vi "Calibration_Estimate X and Y Zoom voltages.vi"(11 "System Type":string="x.voltage") -> (2 "Y.ZOOM_estimated":dbl, 3 "X.ZOOM_estimated":dbl)   [LabVIEW 2012]
uses:
  Custom Controls and Typedefs/FGV_CalibrationKeyParams_Actions.ctl
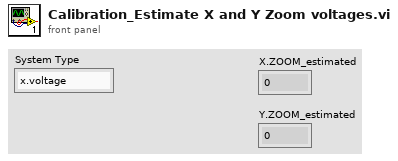
[diagram p1: front panel]
types:
  T1 = typedef "FGV_CalibrationKeyParams_Actions.ctl" = enum16{"Initialize", "Grab From SciScan and Store", "Read Parameters", "ReadGFGValue"}
  T2 = typedef "Calibration Key Param structure.ctl" = cluster{"GFG Variable Name":string, "Data Type":T3, "Value":variant}
  T3 = typedef "VariantType.lvlib/Type.ctl" = enum8{"Invalid Type", "Void", "I8", "I16", "I32", "I64", "U8", "U16", "U32", "U64", "Single Float", "Double Float", "Extended Float", "Single Complex", "Double Complex", "Extended Complex", "Enum U8", "Enum U16", "Enum U32", "Enum U64", "Single Float With Unit", "Double Float With Unit", "Extended Float With Unit", "Single Complex with Unit", "Double Complex with Unit", "Extended Complex with Unit", "Boolean", "String", "Path", "Picture", "Tag", "Array", "Cluster", "Variant", "LV Variant", "Waveform", "Timestamp", "Digital Waveform", "Digital Data", "ExpressData", "Refnum", "External Data", "VI", "Poly VI", "LabVIEW Class Instance", "Fixed Point"}
  T4 = cluster{"Key Parameters Array":T2[], "Key String":string}
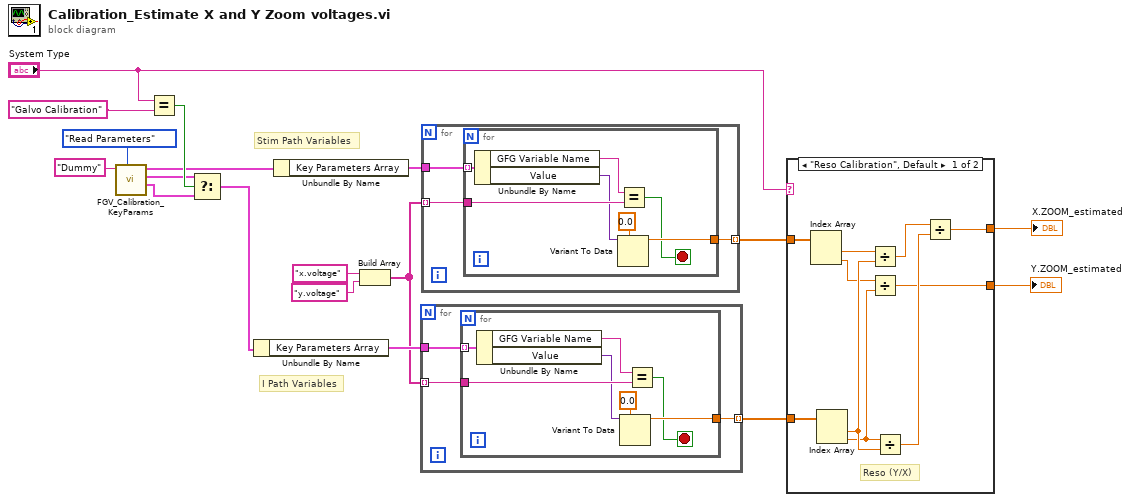
[diagram p0: block diagram]
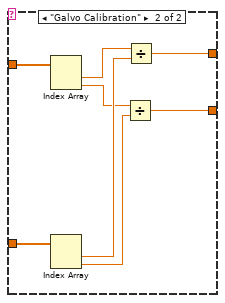
[diagram p2: hidden frame]
diagram:
  # "I Path Variables"
  # "Stim Path Variables"
  n1 = call "FGV_Calibration_KeyParams.vi"("Action"=FGV_CalibrationKeyParams_Actions."Read Parameters", "System Type"="Dummy") -> ("Imaging Reso Key Parameters"=w12:T4, "Imaging Galvo Key Parameters"=w13:T4, "Stimulating Galvo Key Parameters"=w5:T4)  [unwired: 4 in, 3 out]
  n2 = Equal?(x="System Type", y="Galvo Calibration" ("System Type")) -> (x = y?=w16:bool)
  n3 = Select(t=w13, s=w16, f=w12) -> (s? t:f=w6:T4)
  n4 = Unbundle By Name(w6) -> ("Key Parameters Array"=w8:T2[])
  n5 = Unbundle By Name(w5) -> ("Key Parameters Array"=w9:T2[])
  n6 = Build Array("x.voltage" ("System Type"), "y.voltage" ("System Type")) -> (w7:string[])
  n7 = for {
    tunnel: w7 -> [w20] mode=indexing
    tunnel: w8 -> [w21]
    tunnel: [w19] -> w3 mode=indexing
    n8 = for {
      tunnel: w21 -> [w28] mode=indexing
      tunnel: w20 -> [w27]
      tunnel: [w23] -> w19
      stop <- w22 stop-if-true
      n9 = Unbundle By Name(w28) -> ("GFG Variable Name"=w24:string, "Value"=w26:variant)
      n10 = Variant To Data(type=0.0, Variant=w26) -> (data=w23:dbl)  [unwired: 1 in, 1 out]
      n11 = Equal?(x=w24, y=w27) -> (x = y?=w22:bool)
    }
  }
  n12 = for {
    tunnel: w7 -> [w30] mode=indexing
    tunnel: w9 -> [w31]
    tunnel: [w29] -> w4 mode=indexing
    n13 = for {
      tunnel: w31 -> [w38] mode=indexing
      tunnel: w30 -> [w37]
      tunnel: [w33] -> w29
      stop <- w32 stop-if-true
      n14 = Unbundle By Name(w38) -> ("GFG Variable Name"=w34:string, "Value"=w36:variant)
      n15 = Variant To Data(type=0.0, Variant=w36) -> (data=w33:dbl)  [unwired: 1 in, 1 out]
      n16 = Equal?(x=w34, y=w37) -> (x = y?=w32:bool)
    }
  }
  n17 = case shown="\"Reso Calibration\", Default" "System Type" {
    tunnel: [w42 w52] -> w18
    tunnel: [w41 w51] -> w17
    tunnel: w4 -> [w40 w50]
    tunnel: w3 -> [w39 w49]
    frame "Reso Calibration", Default {
      # "Reso (Y/X)"
      n18 = Index Array(array=w40) -> (element #1=w43:dbl, element #2=w44:dbl)  [unwired: 2 in]
      n19 = Index Array(array=w39) -> (element #1=w46:dbl, element #2=w45:dbl)  [unwired: 2 in]
      n20 = Divide(x=w43, y=w46) -> (x/y=w47:dbl)
      n21 = Divide(x=w44, y=w45) -> (x/y=w41:dbl)
      n22 = Divide(x=w45, y=w46) -> (x/y=w48:dbl)
      n23 = Divide(x=w47, y=w48) -> (x/y=w42:dbl)
    }
    frame "Galvo Calibration" {
      n24 = Index Array(array=w50) -> (element #1=w56:dbl, element #2=w54:dbl)  [unwired: 2 in]
      n25 = Index Array(array=w49) -> (element #1=w55:dbl, element #2=w53:dbl)  [unwired: 2 in]
      n26 = Divide(x=w54, y=w53) -> (x/y=w51:dbl)
      n27 = Divide(x=w56, y=w55) -> (x/y=w52:dbl)
    }
  }
  "X.ZOOM_estimated" <- w18
  "Y.ZOOM_estimated" <- w17
